vi "Measurement UI.vi"() -> ()   [LabVIEW 2021, in "Short-Circuit UI.lvlib"]
uses:
  Short-Circuit UI.lvlib
panel:
  in  "MeasGraphs":enum32{"Source & Load Results"}(tab)
  out "Graph-Output Voltage":dbl[](graph) caption="Load Transient"
  out "Graph-Output Current":dbl[](graph) caption="Load Transient"
  out "Display Table":i32(listbox)
  in  "Configurations tab":T1(tab)=enum."Source Config"
  in  "Source delay":dbl=0.005 caption="SOURCE DELAY" format="%.3ps"
  in  "DUT setup time":dbl=1.0 caption="DUT SETUP TIME" format="%.3ps"
  in  "Aperture time":dbl=0.005 caption="APERTURE TIME" format="%.3ps"
  in  "Source current limit":dbl=2.0 caption="CURRENT LIMIT" format="%#_6pA"
  in  "PPSResourceName":refnum<k15> caption="RESOURCE NAME"
  in  "Source sense":i32(ring)=1009 caption="SENSE" items=["Local"=1008, "Remote"=1009]
  in  "Source maximum power":dbl=20.0 caption="MAXIMUM POWER" format="%#_6pW"
  in  "Source Voltage (Vo)":dbl=3.5 caption="SOURCE VOLTAGE" format="%#_6pV"
  in  "Load Voltage Limit":dbl=6.0 caption="VOLTAGE  LIMIT" format="%#_6pV"
  in  "Load voltage limit range":dbl=60.0 caption="VOLTAGE LIMIT RANGE" format="%#_6pV"
  in  "Load Current Level (Io)":dbl=0.1 caption="LOAD CURRENT" format="%#_6pA"
  in  "Load sense":i32(ring)=1009 caption="SENSE" items=["Local"=1008, "Remote"=1009]
  in  "LoadResourceName":refnum<k15> caption="RESOURCE NAME"
  in  "Switch - DMM Relay Name":string="k1" caption="DMM RELAY NAME"
  in  "Switch - Load Relay Name":string="k0" caption="LOAD RELAY NAME"
  in  "SwitchResourceName":refnum<k15> caption="RESOURCE NAME"
  in  "Switch Relay Topology":string(combo)="Configured Topology" caption="RELAY TOPOLOGY"
  in  "DMMResourceName":refnum<k15> caption="RESOURCE NAME"
  in  "DMM Current Range(A)":dbl=14.0 caption="RANGE" format="%#_6pA"
  in  "DMM Resolution":dbl(ring)=5.5 caption="RESOLUTION IN DIGITS" items=["3 1/2"=3.5, "4 1/2"=4.5, "5 1/2"=5.5, "6 1/2"=6.5, "7 1/2"=7.5]
  in  "SC - Trigger Delay (sec)":dbl=5.0 caption="TRIGGER DELAY" format="%.2ps"
  in  "SC - Hold Delay (sec)":dbl=5.0 caption="HOLD DELAY" format="%.2ps"
  out "Load Current":dbl[](array[numeric])
  out "Source Current":dbl[](array[numeric])
  out "Load voltages":dbl[](array[numeric])
  out "Source voltages":dbl[](array[numeric])
  in  "Source resource name":string caption="RESOURCE NAME"
  in  "Load resource name":string caption="RESOURCE NAME"
  in  "DMM resource name":string caption="RESOURCE NAME"
  in  "Switch resource name":string caption="RESOURCE NAME"
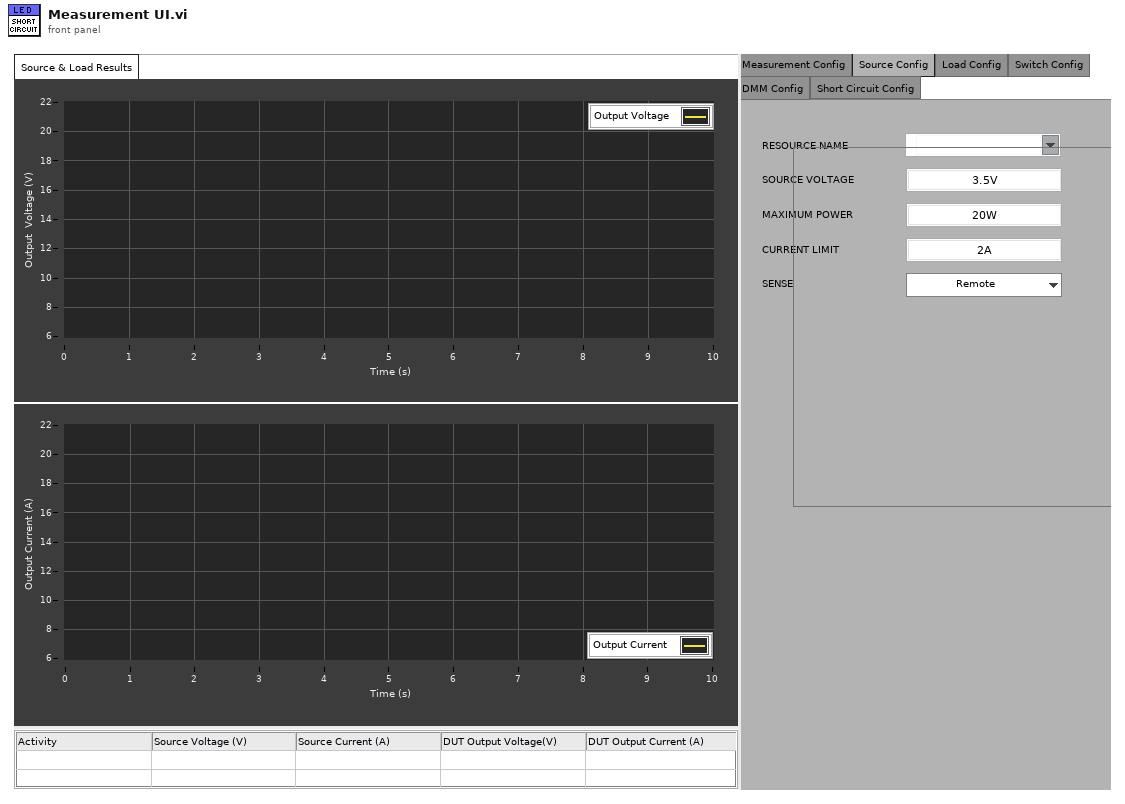
[diagram p1: front panel]
types:
  T1 = enum32{"Measurement Config", "Source Config", "Load Config", "Switch Config", "DMM Config", "Short Circuit Config", "Hidden Controls"}
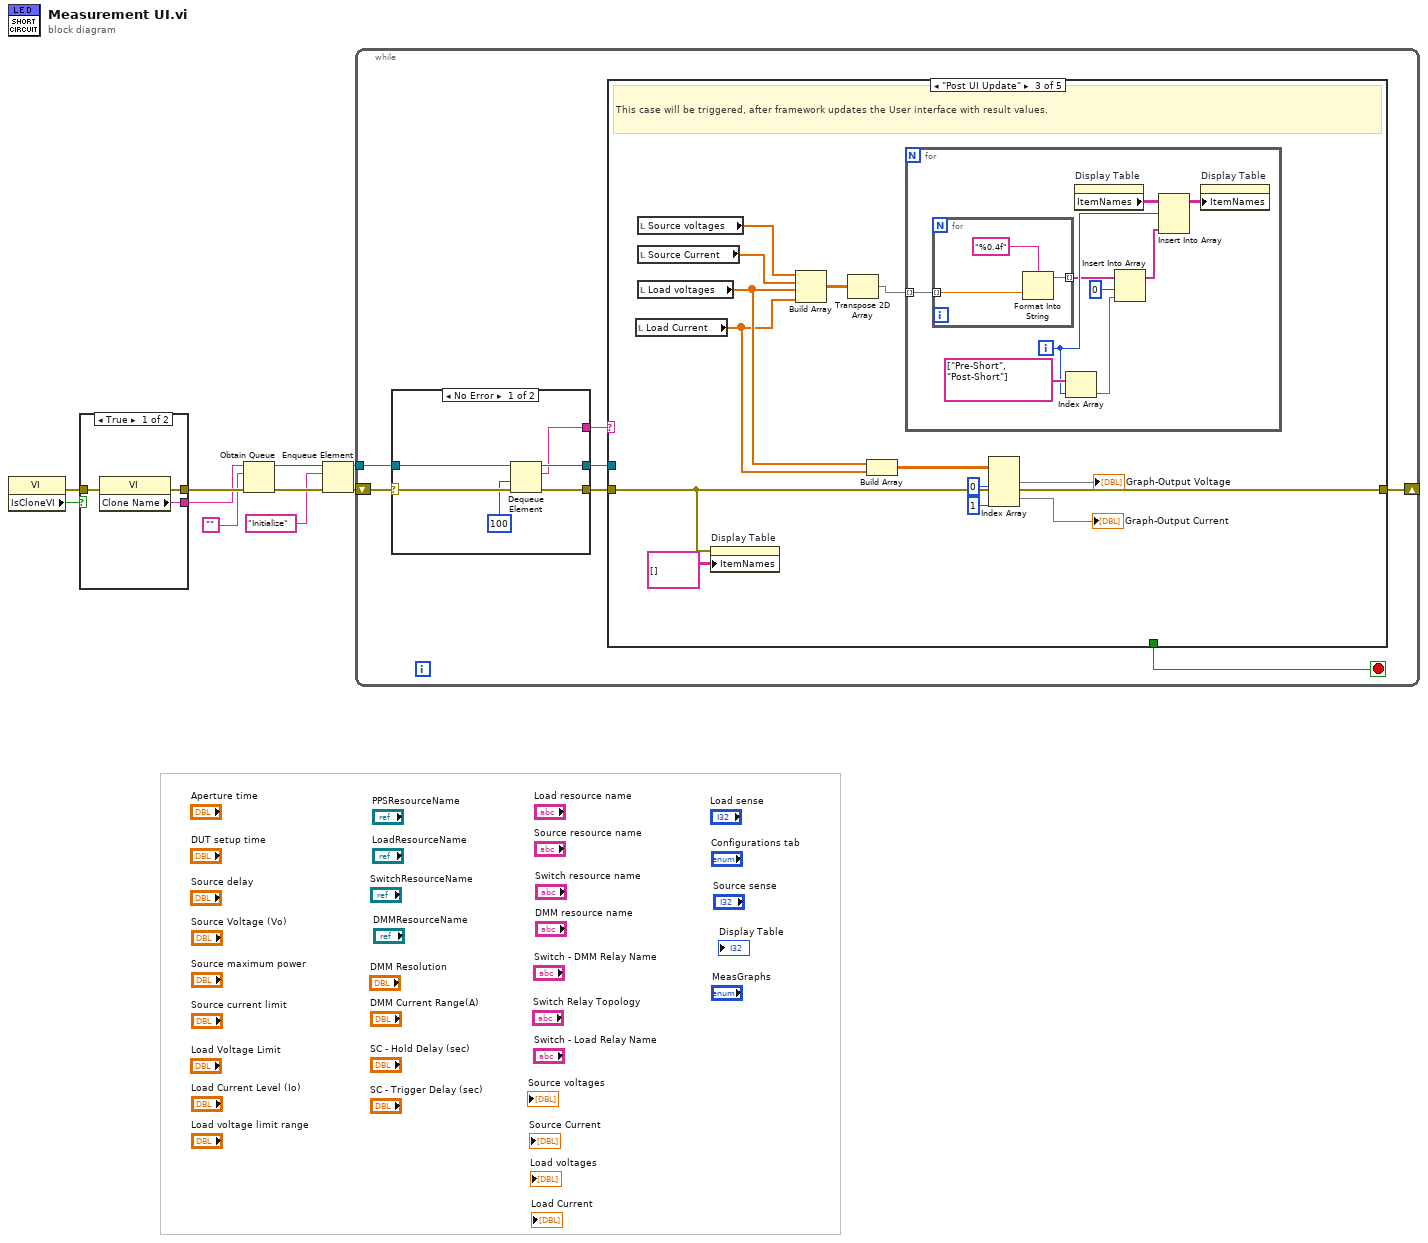
[diagram p0: block diagram]
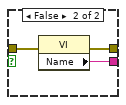
[diagram p2: hidden frame]
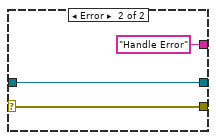
[diagram p3: hidden frame]
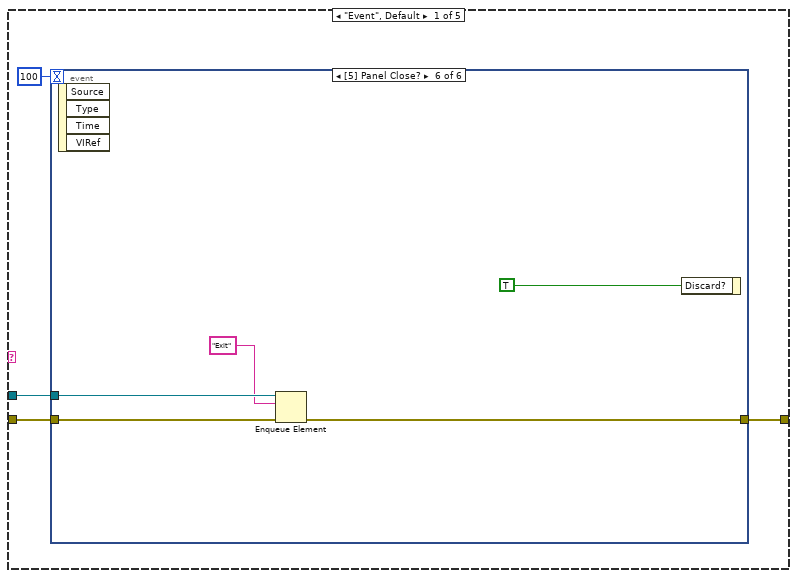
[diagram p4: hidden frame]
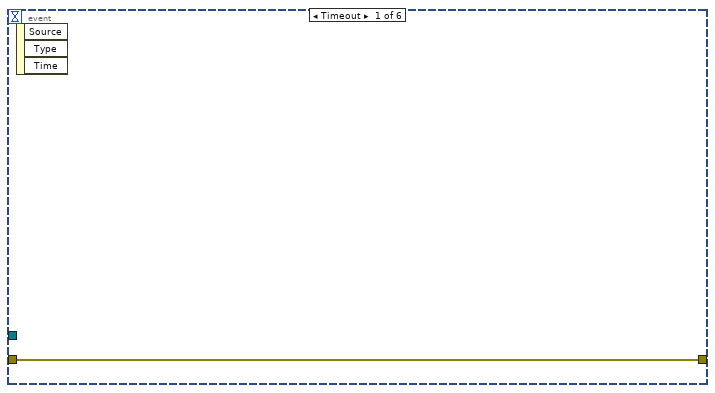
[diagram p5: hidden frame]
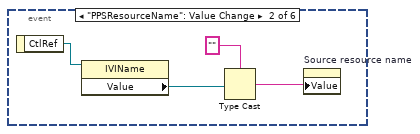
[diagram p6: hidden frame]
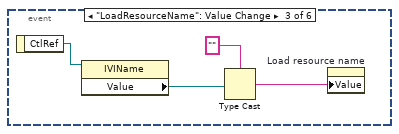
[diagram p7: hidden frame]
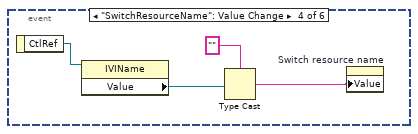
[diagram p8: hidden frame]
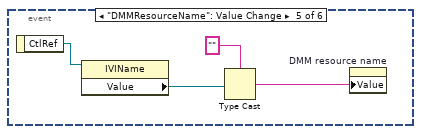
[diagram p9: hidden frame]
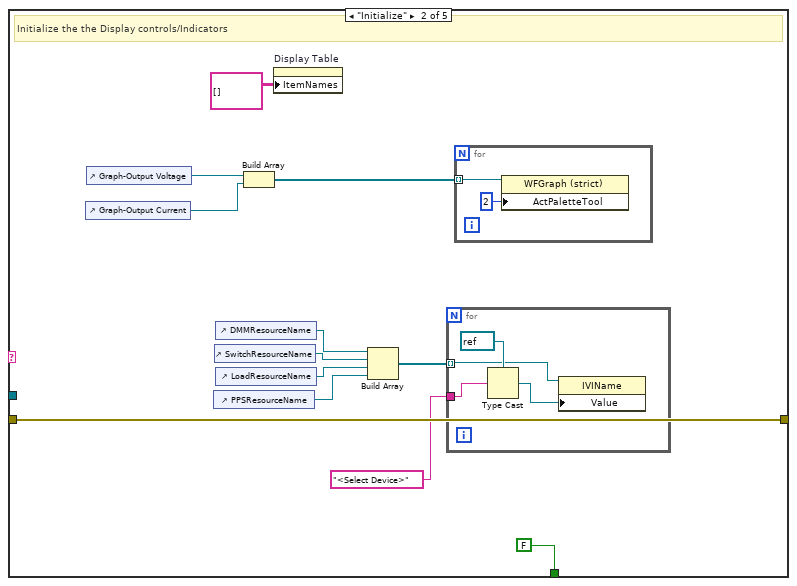
[diagram p10: hidden frame]
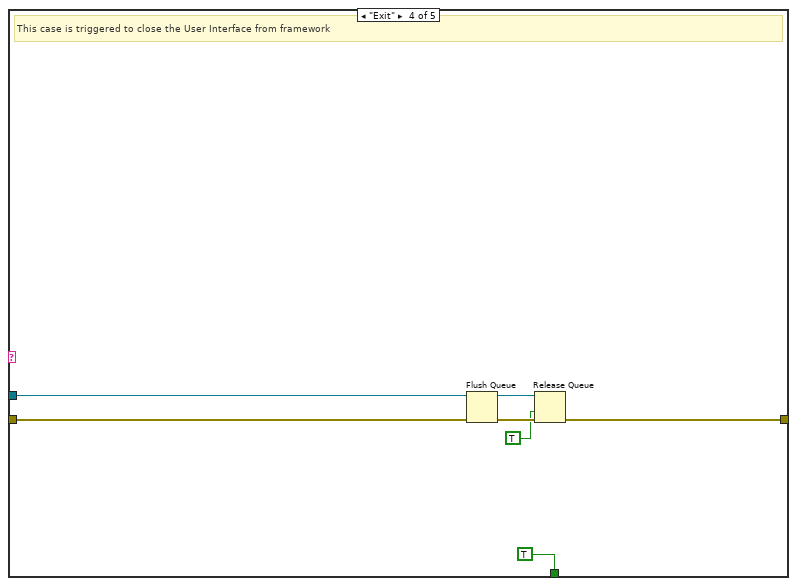
[diagram p11: hidden frame]
diagram:
  n1 = property class="VI"() -> (error out=w1:errorcluster, "IsCloneVI"=w2:bool)  [unwired: 2 in, 1 out]
  n2 = case shown="True" w2 {
    tunnel: [w13 w16] -> w10
    tunnel: [w12 w15] -> w9
    tunnel: w1 -> [w11 w14]
    frame True {
      n3 = property class="VI"(error in=w11) -> (error out=w13:errorcluster, "Clone Name"=w12:string)  [unwired: 1 in, 1 out]
    }
    frame False {
      n4 = property class="VI"(error in=w14) -> (error out=w16:errorcluster, "Name"=w15:string)  [unwired: 1 in, 1 out]
    }
  }
  n5 = Obtain Queue(name (unnamed)=w9, element data type="", error in (no error)=w10) -> (queue out=w6:refnum<queue>, error out=w8:errorcluster)  [unwired: 2 in, 1 out]
  n6 = Enqueue Element(queue=w6, element="Initialize", error in (no error)=w8) -> (queue out=w5:refnum<queue>, error out=w7:errorcluster)  [unwired: 1 in, 1 out]
  n7 = while {
    shift-right: [w18] -> _
    shift-left: w7 -> [w23]
    tunnel: w5 -> [w21]
    stop <- w17 stop-if-true
    n8 = case shown="No Error" w23 {
      selector: w23 -> [w29 w32]
      tunnel: [w28 w32] -> w22
      tunnel: w21 -> [w27 w31]
      tunnel: [w26 w31] -> w20
      tunnel: [w25 "Handle Error"] -> w19
      frame No Error {
        n9 = Dequeue Element(queue=w27, timeout in ms (-1)=100, error in (no error)=w29) -> (queue out=w26:refnum<queue>, element=w25:string, error out=w28:errorcluster)  [unwired: 1 out]
      }
      frame Error {
      }
    }
    n10 = case shown="\"Post UI Update\"" w19 {
      tunnel: w22 -> [w35 w70 w79 w108 w109]
      tunnel: w20 -> [w33 _ _ w106 _]
      tunnel: [w36 w70 w79 w103 w109] -> w18
      tunnel: [_ FALSE _ TRUE _] -> w17
      frame "Event", Default {
        n11 = event shown="[5] Panel Close?" {
          selector: _ -> [_ _ _ _ _ _]
          dyn-events: _ -> [_ _ _ _ _ _]
          timeout: 100 -> [_ _ _ _ _ _]
          tunnel: [w37 _ _ _ _ w56] -> w36
          tunnel: w35 -> [w37 _ _ _ _ w57]
          tunnel: w33 -> [_ _ _ _ _ w55]
          event Timeout {
            n12 = event-data() -> ()  [unwired: 1 in, 3 out]
          }
          event "PPSResourceName": Value Change {
            n13 = event-data() -> ("CtlRef"=w41:refnum<vi>)  [unwired: 1 in]
            n14 = property class="IVIName"(reference=w41) -> ("Value"=w40:refnum<k15>)  [unwired: 1 in, 2 out]
            n15 = Type Cast(type="", x=w40) -> (*(type *) &x=w38:string)
            n16 = property on="Source resource name" class="Str"("Value"=w38) -> ()  [unwired: 2 in, 2 out]
          }
          event "LoadResourceName": Value Change {
            n17 = event-data() -> ("CtlRef"=w45:refnum<vi>)  [unwired: 1 in]
            n18 = property class="IVIName"(reference=w45) -> ("Value"=w44:refnum<k15>)  [unwired: 1 in, 2 out]
            n19 = Type Cast(type="", x=w44) -> (*(type *) &x=w42:string)
            n20 = property on="Load resource name" class="Str"("Value"=w42) -> ()  [unwired: 2 in, 2 out]
          }
          event "SwitchResourceName": Value Change {
            n21 = event-data() -> ("CtlRef"=w49:refnum<vi>)  [unwired: 1 in]
            n22 = property class="IVIName"(reference=w49) -> ("Value"=w48:refnum<k15>)  [unwired: 1 in, 2 out]
            n23 = Type Cast(type="", x=w48) -> (*(type *) &x=w46:string)
            n24 = property on="Switch resource name" class="Str"("Value"=w46) -> ()  [unwired: 2 in, 2 out]
          }
          event "DMMResourceName": Value Change {
            n25 = event-data() -> ("CtlRef"=w53:refnum<vi>)  [unwired: 1 in]
            n26 = property class="IVIName"(reference=w53) -> ("Value"=w52:refnum<k15>)  [unwired: 1 in, 2 out]
            n27 = Type Cast(type="", x=w52) -> (*(type *) &x=w50:string)
            n28 = property on="DMM resource name" class="Str"("Value"=w50) -> ()  [unwired: 2 in, 2 out]
          }
          event Panel Close? {
            n29 = event-data() -> ()  [unwired: 1 in, 4 out]
            n30 = Enqueue Element(queue=w55, element="Exit", error in (no error)=w57) -> (error out=w56:errorcluster)  [unwired: 1 in, 2 out]
            n31 = event-data("Discard?"=TRUE) -> ()  [unwired: 1 in, 1 out]
          }
        }
      }
      frame "Initialize" {
        # "Initialize the the Display controls/Indicators"
        n32 = control-ref of="Graph-Output Current"() -> (w59:refnum<vi>)
        n33 = control-ref of="Graph-Output Voltage"() -> (w60:refnum<vi>)
        n34 = control-ref of="PPSResourceName"() -> (w64:refnum<vi>)
        n35 = control-ref of="SwitchResourceName"() -> (w66:refnum<vi>)
        n36 = control-ref of="DMMResourceName"() -> (w67:refnum<vi>)
        n37 = control-ref of="LoadResourceName"() -> (w65:refnum<vi>)
        n38 = Build Array(w60, w59) -> (w68:refnum<vi>[])
        n39 = property on="Display Table" class="MCListbox (strict)"("ItemNames"=string[][] [] ("Item Names")) -> ()  [unwired: 2 in, 2 out]
        n40 = Build Array(w67, w66, w65, w64) -> (w63:refnum<vi>[])
        n41 = for {
          tunnel: w63 -> [w71] mode=indexing
          tunnel: "<Select Device>" -> [w74]
          n42 = Type Cast(type=refnum<k15> refnum ("Value"), x=w74) -> (*(type *) &x=w72:refnum<k15>)
          n43 = property class="IVIName"(reference=w71, "Value"=w72) -> ()  [unwired: 1 in, 2 out]
        }
        n44 = for {
          tunnel: w68 -> [w76] mode=indexing
          n45 = property class="WFGraph (strict)"(reference=w76, "ActPaletteTool"=2 ("Palette:Active Tool")) -> ()  [unwired: 1 in, 2 out]
        }
      }
      frame "Post UI Update" {
        # "This case will be triggered, after framework updates the User interface with result values."
        n46 = local read "Load Current"() -> (w82:dbl[])
        n47 = local read "Source voltages"() -> (w89:dbl[])
        n48 = local read "Source Current"() -> (w84:dbl[])
        n49 = local read "Load voltages"() -> (w83:dbl[])
        n50 = property on="Display Table" class="MCListbox (strict)"(error in=w79, "ItemNames"=string[][] [] ("Item Names")) -> ()  [unwired: 1 in, 2 out]
        n51 = Build Array(w89, w84, w83, w82) -> (w88:dbl[][])
        n52 = Transpose 2D Array(2D array=w88) -> (transposed array=w81:dbl[][])
        n53 = Build Array(w83, w82) -> (w87:dbl[][])
        n54 = for {
          tunnel: w81 -> [w91] mode=indexing
          i -> [w92]
          n55 = for {
            tunnel: w91 -> [w100] mode=indexing
            tunnel: [w99] -> w90 mode=indexing
            n56 = Format Into String(format string="%0.4f", w100) -> (resulting string=w99:string)  [unwired: 2 in, 1 out]
          }
          n57 = Index Array(array=string[] ["Pre-Short", "Post-Short"], index=w92) -> (element=w93:string)
          n58 = property on="Display Table" class="MCListbox (strict)"() -> ("ItemNames"=w98:string[][])  [unwired: 2 in, 2 out]
          n59 = Insert Into Array(array=w90, index=0, new element=w93) -> (w96:string[])
          n60 = Insert Into Array(array=w98, index (row)=w92, new element=w96) -> (w97:string[][])  [unwired: 1 in]
          n61 = property on="Display Table" class="MCListbox (strict)"("ItemNames"=w97) -> ()  [unwired: 2 in, 2 out]
        }
        n62 = Index Array(array=w87, index (col) #1=0 ("disabled index (col)"), index (row) #2=1 ("disabled index (row)")) -> (element #1=→"Graph-Output Voltage":dbl[], element #2=→"Graph-Output Current":dbl[])  [unwired: 2 in]
      }
      frame "Exit" {
        # "This case is triggered to close the User Interface from framework"
        n63 = Flush Queue(queue=w106, error in (no error)=w108) -> (queue out=w105:refnum<queue>, error out=w104:errorcluster)  [unwired: 1 out]
        n64 = Release Queue(queue=w105, force destroy? (F)=TRUE, error in (no error)=w104) -> (error out=w103:errorcluster)  [unwired: 2 out]
      }
      frame "Handle Error" {
      }
    }
  }
